vi "EIP Unconfigured.vi"(8 "error in (no error)":errorcluster, 11 "Node Ptr":T1 format="%.0x") -> (0 "error out":errorcluster)   [LabVIEW 2011, in "Ethernet IP Custom Device Custom Device.lvlib"]
uses:
  Ethernet IP Custom Device Custom Device.lvlib
  <vilib>/NI Veristand/Custom Device API/Custom Device Item Ref.ctl
  <vilib>/NI Veristand/Custom Device API/Custom Device Channel.ctl
  <vilib>/NI Veristand/Custom Device API/Custom Device Channel Type.ctl
  Ethernet IP Global Strings.vi
  <vilib>/NI Veristand/Custom Device API/Get Item Property (Path).vi
  Ethernet IP Global Tag Array.vi
  Ethernet IP Global GUIDs.vi
  <vilib>/NI Veristand/Custom Device API/Custom Device API.lvlib
panel:
  out "Status Information":string
  out "Description":string
  in  "Config Done":bool
  out "Tags not Imported":string
  in  "Unconfigured Tags":i32(listbox)
  in  "Header":cluster{"Section Name":string}={"Section Name"="Custom Device Item Settings"}
  out "Name":string
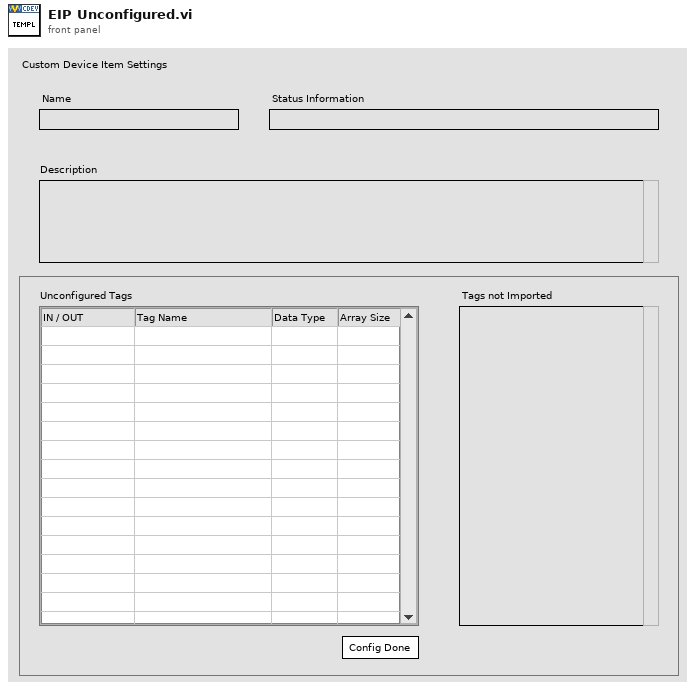
[diagram p1: front panel]
types:
  T1 = typedef "Custom Device API.lvlib/Custom Device Item Ref.ctl" = u64
  T2 = typedef "Custom Device API.lvlib/Custom Device Item Info.ctl" = cluster{"Name":string, "Is Channel":bool, "GUID":string}
  T3 = typedef "Ethernet IP Custom Device Custom Device.lvlib/L5K Internal Data.ctl" = cluster{"L5K Entire String":string, "L5K Extractred String Array":string[], "IP address from CommPath":string, "Configured Tags":T4[], "Data String Array":string[], "Unconfigured Tags":T4[], "# Tags":i32}
  T4 = typedef "Ethernet IP Custom Device Custom Device.lvlib/L5K Tag.ctl" = cluster{"Tag Name":string, "Data Type":T5, "Data Type String":string, "Array Size":i32, "Description":string, "Input?":bool, "Channel Name":string}
  T5 = typedef "Ethernet IP Custom Device Custom Device.lvlib/L5K Data Types.ctl" = enum16{"SINT", "INT", "DINT", "REAL", "BOOL"}
  T6 = typedef "Custom Device API.lvlib/Custom Device Channel.ctl" = cluster{"Type":T7, "Units":string, "Default Value":dbl, "Faultable":bool, "Scalable":bool}
  T7 = typedef "Custom Device API.lvlib/Custom Device Channel Type.ctl" = enum16{"Input", "Output"}
  T8 = typedef "Custom Device API.lvlib/Custom Device Commands.ctl" = enum16{"Default", "Item renamed", "Shutdown", "Dynamic button pressed"}
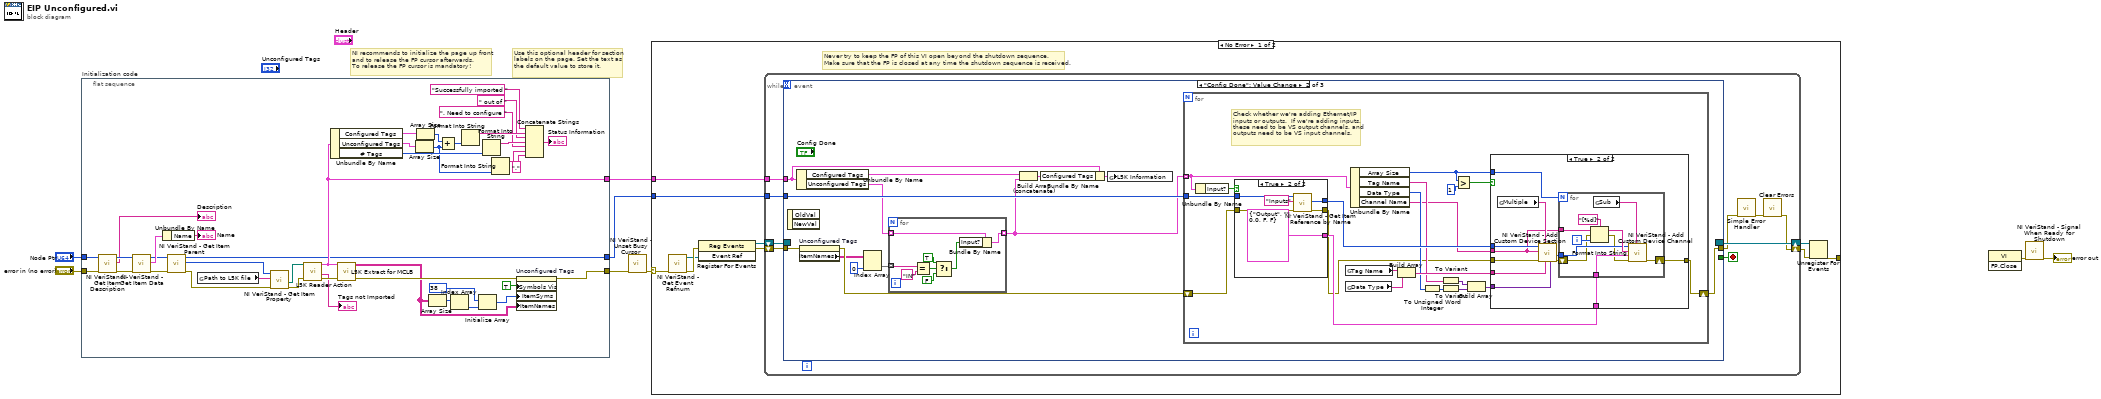
[diagram p0: block diagram]
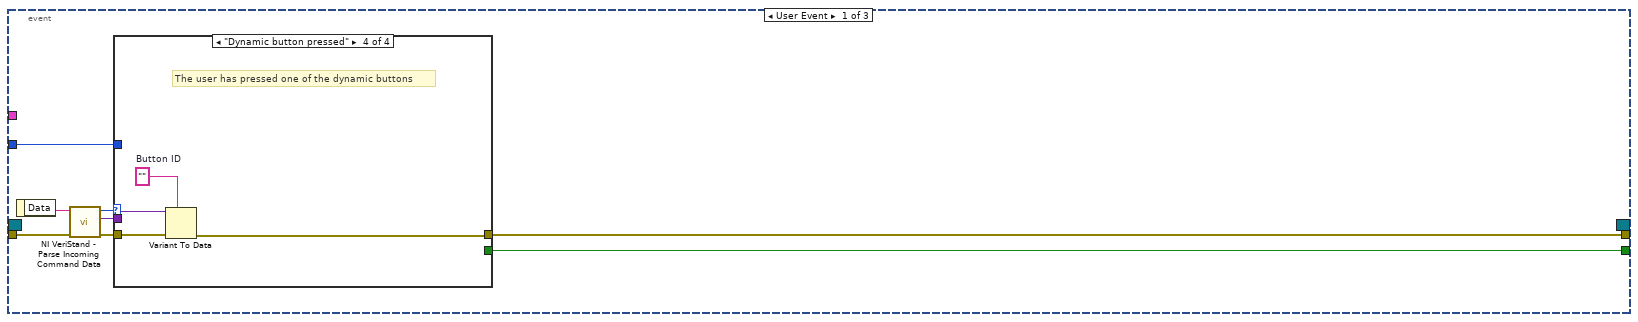
[diagram p2: hidden frame]
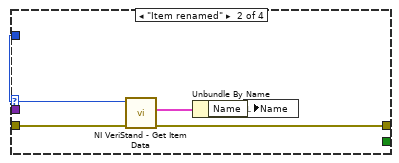
[diagram p4: hidden frame]
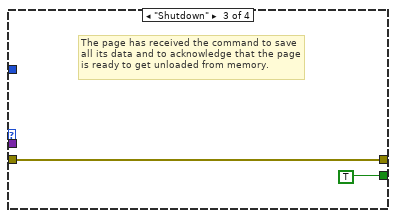
[diagram p5: hidden frame]
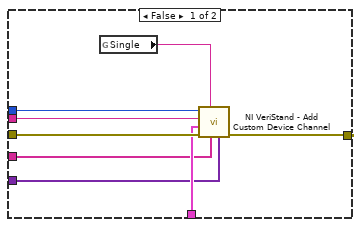
[diagram p6: hidden frame]
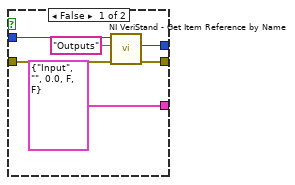
[diagram p7: hidden frame]
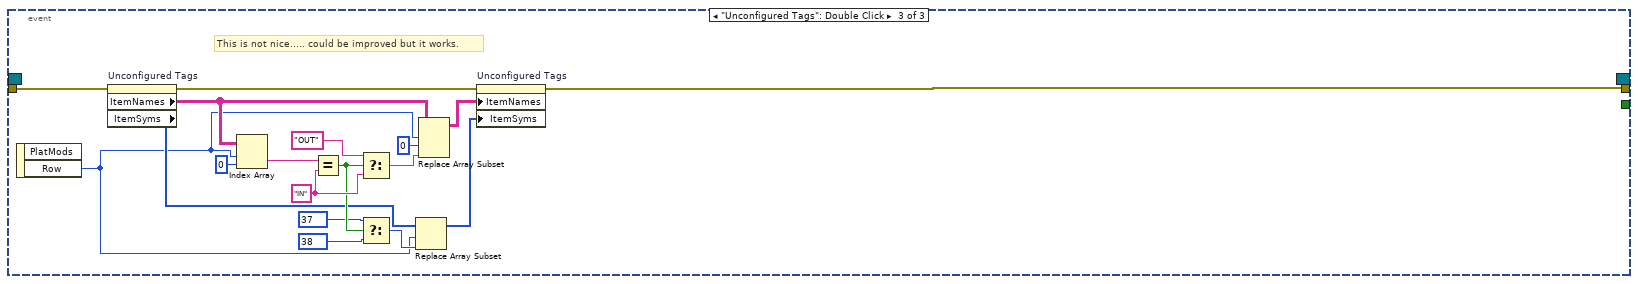
[diagram p8: hidden frame]
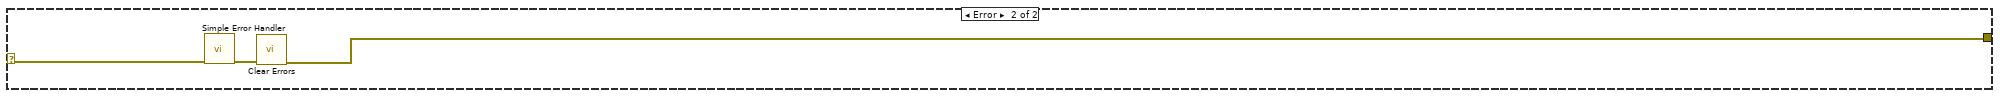
[diagram p9: hidden frame]
diagram:
  # "Use this optional header for section labels on the page. Set the text as the default value to store it."
  # "NI recommends to initialize the page up front\nand to release the FP cursor afterwards.\nTo release the FP cursor is mandatory!"
  n1 = flat-sequence "Initialization code" {
    tunnel: "error in (no error)" -> [w25]
    tunnel: "Node Ptr" -> [w28]
    tunnel: [w40] -> w5
    tunnel: [w30] -> w2
    tunnel: [w37] -> w1
    frame #0 {
      n2 = call <vilib>:"NI VeriStand - Get Item Description.vi"("error in (no error)"=w25, "Item Ref in"=w28) -> ("error out"=w26:errorcluster, "Description"=→"Description":string, "Item Ref out"=w27:T1)  [unwired: 7 out]
      n3 = call <vilib>:"NI VeriStand - Get Item Data.vi"("error in (no error)"=w26, "Item Ref in"=w27) -> ("error out"=w36:errorcluster, "Item Info"=w48:T2, "Item Ref out"=w31:T1)  [unwired: 7 out]
      n4 = Unbundle By Name(w48) -> ("Name"=→"Name":string)
      n5 = call <vilib>:"NI VeriStand - Get Item Parent.vi"("error in (no error)"=w36, "Item Ref in"=w31) -> ("error out"=w32:errorcluster, "Parent Ref"=w34:T1, "Item Ref out"=w30:T1)  [unwired: 6 in, 1 out]
      n6 = global read "Ethernet IP Global Strings.vi" "Path to L5K file"() -> (w35:string)
      n7 = call-poly <vilib>:"NI VeriStand - Get Item Property.vi"("error in (no error)"=w32, "Property Name"=w35, "Item Ref in"=w34) -> ("error out"=w33:errorcluster, "Value"=w29:path)  [unwired: 5 in, 2 out]
      n8 = call "L5K Reader Action.vi"("error in"=w33, "L5K File Path"=w29) -> ("error out"=w39:errorcluster, "Import Error"=→"Tags not Imported":string, "L5K Information"=w37:T3)  [unwired: 7 in]
      n9 = Unbundle By Name(w37) -> ("Configured Tags"=w22:T4[], "Unconfigured Tags"=w21:T4[], "# Tags"=w15:i32)
      n10 = call "L5K Extract for MCLB.vi"("error in"=w39, "L5K Information"=w37) -> ("error out"=w47:errorcluster, "Tag Info for MCLB"=w41:string[][])  [unwired: 8 in]
      n11 = Array Size(array=w21) -> (size(s)=w12:i32)
      n12 = Array Size(array=w22) -> (size(s)=w20:i32)
      n13 = Array Size(array=w41) -> (size(s)=w45:i32[])
      n14 = Add(x=w20, y=w12) -> (x+y=w19:i32)
      n15 = Index Array(array=w45) -> (element=w44:i32)  [unwired: 1 in]
      n16 = Format Into String(w19) -> (resulting string=w17:string)  [unwired: 3 in, 1 out]
      n17 = Initialize Array(38, w44) -> (w42:i32[])
      n18 = Format Into String(w15) -> (resulting string=w14:string)  [unwired: 3 in, 1 out]
      n19 = Format Into String(w12) -> (resulting string=w11:string)  [unwired: 3 in, 1 out]
      n20 = property on="Unconfigured Tags" class="MCListbox (strict)"(error in=w47, "Symbols Vis"=TRUE ("Visible Items:Symbols Visible"), "ItemSyms"=w42, "ItemNames"=w41) -> (error out=w40:errorcluster)  [unwired: 1 in, 1 out]
      n21 = Concatenate Strings("Successfully imported " ("string"), w17, " out of " ("string"), w14, ". Need to configure " ("string"), w11, ".") -> (→"Status Information":string)
    }
  }
  n22 = call <vilib>:"NI VeriStand - Unset Busy Cursor.vi"("error in (no error)"=w5) -> ("error out"=w4:errorcluster)  [unwired: 10 out]
  n23 = case shown="No Error" w4 {
    selector: w4 -> [w50 w191]
    tunnel: [w55 w189] -> _
    tunnel: w2 -> [w51 _]
    tunnel: w1 -> [w49 _]
    frame No Error {
      # "Never try to keep the FP of this VI open beyond the shutdown sequence.\nMake sure that the FP is closed at any time the shutdown sequence is received."
      n24 = call <vilib>:"NI VeriStand - Get Event Refnum.vi"("error in (no error)"=w50) -> ("error out"=w58:errorcluster, "Event Ref"=w54:refnum<user-event>)  [unwired: 9 out]
      n25 = register-events(error in=w58, w54) -> (reference out=w52:refnum<event-registration>, error out=w53:errorcluster)  [unwired: 1 in]
      n26 = while {
        tunnel: w51 -> [w63]
        shift-right: [w60] -> w56
        shift-left: w53 -> [w66]
        shift-right: [w67] -> w57
        shift-left: w52 -> [w65]
        tunnel: w49 -> [w59]
        stop <- w64 stop-if-true
        n27 = event shown="[1] \"Config Done\": Value Change" {
          selector: w65 -> [_ _ _]
          dyn-events: [_ _ _] -> w67
          timeout: _ -> [_ _ _]
          tunnel: w66 -> [w75 w99 w172]
          tunnel: [w71 _ _] -> w64
          tunnel: [w70 w90 w171] -> w62
          tunnel: w63 -> [w69 w98 _]
          tunnel: w59 -> [_ w94 _]
          event User Event {
            n28 = event-data() -> ("Data"=w74:string)  [unwired: 1 out]
            n29 = call <vilib>:"NI VeriStand - Parse Incoming Command Data.vi"("error in (no error)"=w75, "Incoming data"=w74) -> ("error out"=w73:errorcluster, "Outgoing data"=w68:variant, "Action"=w72:T8)  [unwired: 7 out]
            n30 = case shown="\"Dynamic button pressed\"" w72 {
              tunnel: w73 -> [w76 w81 w82 w87]
              tunnel: [_ _ TRUE _] -> w71
              tunnel: [w76 w78 w82 w84] -> w70
              tunnel: w69 -> [_ w80 _ _]
              tunnel: w68 -> [_ _ _ w86]
              frame "Default", Default {
              }
              frame "Item renamed" {
                n31 = call <vilib>:"NI VeriStand - Get Item Data.vi"("error in (no error)"=w81, "Item Ref in"=w80) -> ("error out"=w78:errorcluster, "Item Info"=w79:T2)  [unwired: 8 out]
                n32 = Unbundle By Name(w79) -> ("Name"=w77:string)
                n33 = local write "Name"(w77) -> ()
              }
              frame "Shutdown" {
                # "The page has received the command to save all its data and to acknowledge that the page is ready to get unloaded from memory."
              }
              frame "Dynamic button pressed" {
                w85 = ""  # Button ID
                # "The user has pressed one of the dynamic buttons"
                n34 = Variant To Data(error in=w87, type=w85, Variant=w86) -> (error out=w84:errorcluster)  [unwired: 1 out]
              }
            }
          }
          event "Config Done": Value Change {
            n35 = event-data() -> ()  [unwired: 3 out]
            n36 = Unbundle By Name(w94) -> ("Configured Tags"=w89:T4[], "Unconfigured Tags"=w88:T4[])
            n37 = property on="Unconfigured Tags" class="MCListbox (strict)"(error in=w99) -> (error out=w97:errorcluster, "ItemNames"=w96:string[][])  [unwired: 1 in, 1 out]
            n38 = Index Array(array=w96, index (col)=0 ("disabled index (col)")) -> (element=w95:string[])  [unwired: 1 in]
            n39 = for {
              tunnel: w95 -> [w104] mode=indexing
              tunnel: w88 -> [w103] mode=indexing
              tunnel: [w101] -> w91 mode=indexing
              n40 = Equal?(x=w104, y="IN") -> (x = y?=w107:bool)
              n41 = Select(t=TRUE, s=w107, f=FALSE) -> (s? t:f=w102:bool)
              n42 = Bundle By Name(cluster=w103, "Input?"=w102) -> (w101:T4)
            }
            n43 = Build Array (concatenate)(w89, w91) -> (w92:T4[])
            n44 = Bundle By Name(cluster=w94, "Configured Tags"=w92) -> (w93:T3)
            n45 = global write "Ethernet IP Global Tag Array.vi" "L5K Information"(w93) -> ()
            n46 = for {
              tunnel: w98 -> [w119]
              shift-right: [w117] -> w90
              shift-left: w97 -> [w111]
              tunnel: w91 -> [w113] mode=indexing
              # "Check whether we're adding Ethernet/IP\ninputs or outputs.  If we're adding inputs,\nthese need to be VS output channels, and\noutputs need to be VS input channels."
              n47 = Unbundle By Name(w113) -> ("Input?"=w116:bool)
              n48 = case shown="True" w116 {
                tunnel: [T6 {"Type"=enum."Input", "Units"="", "Default Value"=0.0, "Faultable"=FALSE, "Scalable"=FALSE} ("Channel") T6 {"Type"=enum."Output", "Units"="", "Default Value"=0.0, "Faultable"=FALSE, "Scalable"=FALSE} ("Channel")] -> w129
                tunnel: w119 -> [w163 w169]
                tunnel: [w161 w168] -> w118
                tunnel: w111 -> [w160 w166]
                tunnel: [w159 w165] -> w110
                frame False {
                  n49 = call <vilib>:"NI VeriStand - Get Item Reference by Name.vi"("error in (no error)"=w160, "Item Name"="Outputs", "Parent Ref in"=w163) -> ("error out"=w159:errorcluster, "Item Ref"=w161:T1)  [unwired: 5 in, 2 out]
                }
                frame True {
                  n50 = call <vilib>:"NI VeriStand - Get Item Reference by Name.vi"("error in (no error)"=w166, "Item Name"="Inputs", "Parent Ref in"=w169) -> ("error out"=w165:errorcluster, "Item Ref"=w168:T1)  [unwired: 5 in, 2 out]
                }
              }
              n51 = global read "Ethernet IP Global Strings.vi" "Tag Name"() -> (w121:string)
              n52 = global read "Ethernet IP Global Strings.vi" "Data Type"() -> (w120:string)
              n53 = Unbundle By Name(w113) -> ("Array Size"=w114:i32, "Tag Name"=w112:string, "Data Type"=w115:T5, "Channel Name"=w109:string)
              n54 = Build Array(w121, w120) -> (w124:string[])
              n55 = To Unsigned Word Integer(number=w115) -> (unsigned 16bit integer=w123:u16)
              n56 = To Variant(anything=w112) -> (Variant=w122:variant)
              n57 = To Variant(anything=w123) -> (Variant=w126:variant)
              n58 = Greater?(x=w114, y=1) -> (0:w127:bool)
              n59 = Build Array(w122, w126) -> (w125:variant[])
              n60 = case shown="True" w127 {
                tunnel: w110 -> [w137 w146]
                tunnel: w129 -> [w136 w143]
                tunnel: w109 -> [w130 w139]
                tunnel: w125 -> [w134 w148]
                tunnel: w124 -> [w135 w147]
                tunnel: w118 -> [w133 w142]
                tunnel: [w131 w140] -> w117
                tunnel: w114 -> [_ w138]
                frame False {
                  n61 = global read "Ethernet IP Global GUIDs.vi" "Single"() -> (w132:string)
                  n62 = call <vilib>:"NI VeriStand - Add Custom Device Channel.vi"("Property Values"=w134, "Property names"=w135, "GUID (Default Channel)"=w132, "error in (no error)"=w137, "Channel"=w136, "Channel Name"=w130, "Parent Ref in"=w133) -> ("error out"=w131:errorcluster)  [unwired: 1 in, 3 out]
                }
                frame True {
                  n63 = global read "Ethernet IP Global GUIDs.vi" "Multiple"() -> (w141:string)
                  n64 = call <vilib>:"NI VeriStand - Add Custom Device Section.vi"("Property Values"=w148, "Property names"=w147, "GUID (Default Section)"=w141, "error in (no error)"=w146, "Section Name"=w139, "Parent Ref in"=w142) -> ("error out"=w144:errorcluster, "Section Ptr"=w145:T1)  [unwired: 2 in, 2 out]
                  n65 = for {
                    N: w138 -> [_]
                    tunnel: w145 -> [w155]
                    tunnel: w143 -> [w154]
                    shift-right: [w152] -> w140
                    shift-left: w144 -> [w150]
                    tunnel: w139 -> [w151]
                    i -> [w158]
                    n66 = Format Into String(format string="[%d]", initial string=w151, error in=w150, w158) -> (resulting string=w156:string, error out=w149:errorcluster)
                    n67 = global read "Ethernet IP Global GUIDs.vi" "Sub"() -> (w153:string)
                    n68 = call <vilib>:"NI VeriStand - Add Custom Device Channel.vi"("GUID (Default Channel)"=w153, "error in (no error)"=w149, "Channel"=w154, "Channel Name"=w156, "Parent Ref in"=w155) -> ("error out"=w152:errorcluster)  [unwired: 3 in, 3 out]
                  }
                }
              }
            }
          }
          event "Unconfigured Tags": Double Click {
            w186 = "IN" ("y")
            # "This is not nice..... could be improved but it works."
            n69 = event-data() -> ("Row"=w173:i32)  [unwired: 2 out]
            n70 = property on="Unconfigured Tags" class="MCListbox (strict)"(error in=w172) -> (error out=w181:errorcluster, "ItemNames"=w180:string[][], "ItemSyms"=w176:i32[])  [unwired: 1 in, 1 out]
            n71 = Index Array(array=w180, index (row)=w173, index (col)=0 ("disabled index (col)")) -> (element=w187:string)
            n72 = Equal?(x=w187, y=w186) -> (x = y?=w184:bool)
            n73 = Select(t="OUT" ("y"), s=w184, f=w186) -> (s? t:f=w179:string)
            n74 = Select(t=37, s=w184, f=38) -> (s? t:f=w175:i32)
            n75 = Replace Array Subset(array=w176, new element=w175, index=w173) -> (w174:i32[])
            n76 = Replace Array Subset(array=w180, new element=w179, index (row)=w173, index (col)=0 ("disabled index (col)")) -> (w177:string[][])
            n77 = property on="Unconfigured Tags" class="MCListbox (strict)"(error in=w181, "ItemNames"=w177, "ItemSyms"=w174) -> (error out=w171:errorcluster)  [unwired: 1 in, 1 out]
          }
        }
        n78 = call <vilib>:"Simple Error Handler.vi"("error in (no error)"=w62) -> ("error out"=w61:errorcluster)  [unwired: 1 in, 7 out]
        n79 = call <vilib>:"Clear Errors.vi"("error in (no error)"=w61) -> ("error out"=w60:errorcluster)  [unwired: 6 out]
      }
      n80 = Unregister For Events(event registration refnum=w57, error in=w56) -> (error out=w55:errorcluster)
    }
    frame Error {
      n81 = call <vilib>:"Simple Error Handler.vi"("error in (no error)"=w191) -> ("error out"=w190:errorcluster)  [unwired: 1 in, 7 out]
      n82 = call <vilib>:"Clear Errors.vi"("error in (no error)"=w190) -> ("error out"=w189:errorcluster)  [unwired: 6 out]
    }
  }
  n83 = invoke class="VI" method="FP.Close"() -> (error out=w8:errorcluster)  [unwired: 3 in, 2 out]
  n84 = call <vilib>:"NI VeriStand - Signal When Ready for Shutdown.vi"("error in (no error)"=w8) -> ("error out"=→"error out":errorcluster)  [unwired: 10 out]
